vi "valve_VCH.vi"(4 "ZB01 (F)":bool, 6 "XB24 (F)":bool, 7 "Alarm":bool[](array[boolean])=[FALSE, FALSE], 10 "Z_control":T5={"Z_HSw"=1, "Z_HSetState"=enum."on (closed)", "Z_ASetState"=enum."on (closed)", "Z_DSetState"=enum."on (closed)"}, 11 "valve_VCH_in":refnum<class "valve_VCH.lvclass">) -> (1 "YB":bool[](array[boolean]), 2 "Z_out":T1={"Z_Source"=enum."local disabled", "Z_SetState"=enum."initialization", "Z_State"=enum."initialization", "Z_State_T"=0, "ZM_State"=enum."initialization", "ZM_State_T"=0, "ALR  L1"=FALSE, "ALR  L2"=FALSE, "HH_run"=0}, 3 "valve_VCH_in 2":refnum<class "valve_VCH.lvclass">)   [LabVIEW 2019, in "valve_VCH.lvclass"]
uses:
  valve_VCH.lvclass
  ctl/Z_control_VCH.ctl
  ctl/Z_State_VCH.ctl
  ctl/Z.ctl
  Heating/ctl/Z_source.ctl
  ctl/ZM_State_VCH.ctl
  valve_VCH.lvclass/valve_VCH.ctl
  ZM_state/valve_VCH_ZM_state.lvclass/valve_VCH_ZM_state.ctl
  Z_state/valve_VCH_Z_state.lvclass/valve_VCH_Z_state.ctl
  Sequence/State/State.lvclass/State.ctl
  Sequence/State/Read T (ms).vi
  Z_state/valve_VCH_Z_state.lvclass
  D:/my_projects/projects/Algorithms/Labview/19/Sequence/State/State.lvclass
  ZM_state/valve_VCH_ZM_state.lvclass
  Sequence/State/Step.vi
  Valves.lvlib
  Heating/Heating.lvlib
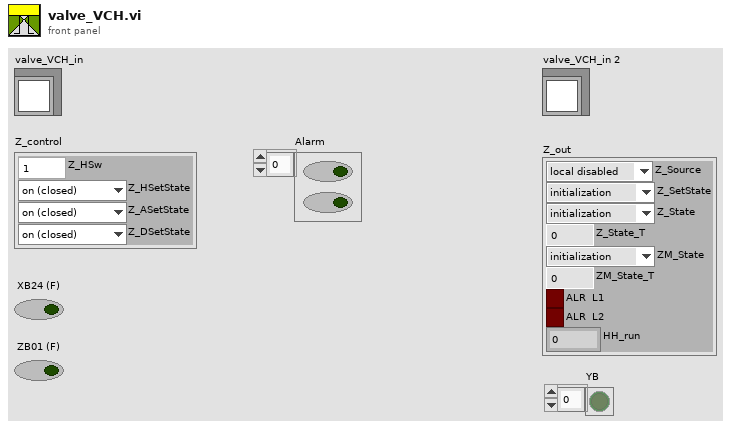
[diagram p1: front panel]
types:
  T1 = typedef "Valves.lvlib/Z.ctl" = cluster{"Z_Source":T2, "Z_SetState":T3, "Z_State":T3, "Z_State_T":u32, "ZM_State":T4, "ZM_State_T":u32, "ALR  L1":bool, "ALR  L2":bool, "HH_run":i32}
  T2 = typedef "Heating.lvlib/Z_source.ctl" = enum8{"initialize", "local disabled", "local hand", "hand", "auto", "dist"}
  T3 = typedef "Valves.lvlib/Z_State_VCH.ctl" = enum8{"initialization", "alarm", "disabled", "not ready", "closed ready", "reserv", "reserv1", "reserv2", "reserv3", "check", "on min", "open", "on (closed)"}
  T4 = typedef "Valves.lvlib/ZM_State_VCH.ctl" = enum8{"initialization", "closed", "big_pause", "little_pause", "open", "close_cmd"}
  T5 = typedef "Valves.lvlib/Z_control_VCH.ctl" = cluster{"Z_HSw":u8, "Z_HSetState":T3, "Z_ASetState":T3, "Z_DSetState":T3}
  T6 = cluster{"Z_Source":T2, "Z_Set_State":T3, "ZM_State":T4}
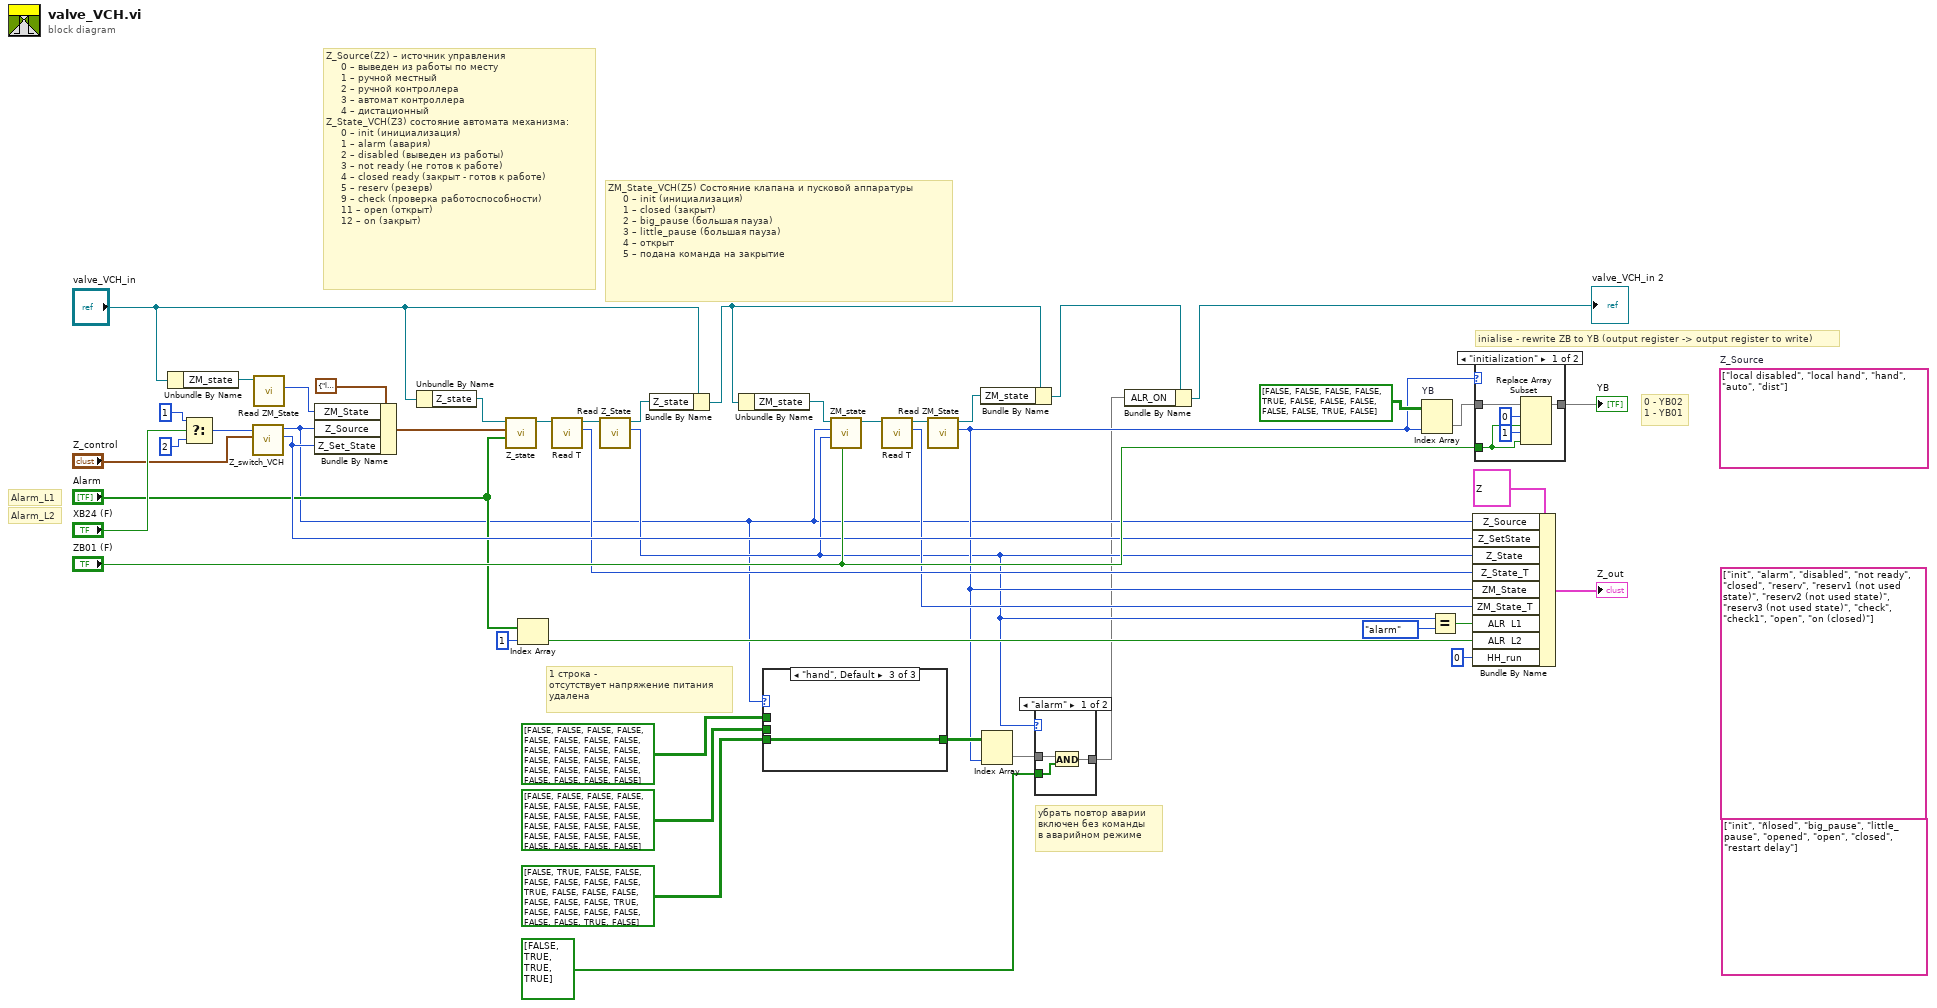
[diagram p0: block diagram]
diagram:
  (unwired) string[] ["init", "alarm", "disabled", "not ready", "closed", "reserv", "reserv1 (not used state)", "reserv2 (not used state)", "reserv3 (not used state)", "check", "check1", "open", "on (closed)"]
  (unwired) string[] ["local disabled", "local hand", "hand", "auto", "dist"]  # Z_Source
  (unwired) string[] ["init", "ñlosed", "big_pause", "little_pause", "opened", "open", "closed", "restart delay"]
  # "Alarm_L2"
  # "Alarm_L1"
  # "inialise - rewrite ZB to YB (output register -> output register to write)"
  # "0 - YB02\n1 - YB01"
  # "1 строка - \nотсутствует напряжение питания\nудалена"
  # "убрать повтор аварии\nвключен без команды\nв аварийном режиме"
  # "Z_Source(Z2) – источник управления\n     0 – выведен из работы по месту\n     1 – ручной местный\n     2 – ручной контроллера\n     3 – автомат контроллера\n     4 – дистационный\nZ_State_VCH(Z3) состояние автомата механизма:\n     0 – init (инициализация)\n     1 – alarm (авария)\n     2 – disabled (выведен из работы)\n     3 – not ready (не готов к работе)\n     4 – closed ready (закрыт - готов к работе)\n     5 – reserv (резерв)\n     9 – check (проверка работоспособности)\n     11 – open (открыт)\n     12 – on (закрыт)"
  # "ZM_State_VCH(Z5) Состояние клапана и пусковой аппаратуры\n     0 – init (инициализация)\n     1 – сlosed (закрыт)\n     2 – big_pause (большая пауза)\n     3 – little_pause (большая пауза)\n     4 – открыт\n     5 – подана команда на закрытие"
  n1 = Unbundle By Name("valve_VCH_in") -> ("ZM_state"=w11:refnum<class "valve_VCH_ZM_state.lvclass">)
  n2 = Select(t=u32 1, s="XB24 (F)", f=u32 2) -> (s? t:f=w43:u32)
  n3 = call "Z_switch_VCH.vi"("Z"="Z_control", "Z_LSw (2-auto)"=w43) -> ("Z_SetState"=w31:T3, "Z_Source"=w7:T2)  [unwired: 8 in]
  n4 = call "Read ZM_State.vi"("valve_VCH_ZM_state in"=w11) -> ("ZM_State_VCH"=w10:T4)  [unwired: 9 in, 1 out]
  n5 = Bundle By Name(cluster=T6 {"Z_Source"=enum."local disabled", "Z_Set_State"=enum."initialization", "ZM_State"=enum."initialization"} ("Z_In"), "ZM_State"=w10, "Z_Source"=w7, "Z_Set_State"=w31) -> (w23:T6)
  n6 = Unbundle By Name("valve_VCH_in") -> ("Z_state"=w3:refnum<class "valve_VCH_Z_state.lvclass">)
  n7 = call "Z_state.vi"("Alarm"="Alarm", "Z_In"=w23, "Z_state in"=w3) -> ("Z_state out"=w20:refnum<class "valve_VCH_Z_state.lvclass">)  [unwired: 8 in]
  n8 = Index Array(array="Alarm", index=1) -> (element=w26:bool)
  n9 = call "Read T.vi"("valve_VCH_Z_state in"=w20) -> ("T (ms)"=w21:u32, "valve_VCH_Z_state out"=w19:refnum<class "valve_VCH_Z_state.lvclass">)  [unwired: 9 in]
  n10 = call "Read Z_State.vi"("valve_VCH_Z_state in"=w19) -> ("Z_State_VCH"=w8:T3, "valve_VCH_Z_state out"=w18:refnum<class "valve_VCH_Z_state.lvclass">)  [unwired: 9 in]
  n11 = Bundle By Name(cluster="valve_VCH_in", "Z_state"=w18) -> (w13:refnum<class "valve_VCH.lvclass">)
  n12 = Unbundle By Name(w13) -> ("ZM_state"=w2:refnum<class "valve_VCH_ZM_state.lvclass">)
  n13 = case shown="\"hand\", Default" w7 {
    tunnel: bool[][] [[FALSE, FALSE, FALSE, FALSE, FALSE, FALSE], [FALSE, FALSE, FALSE, FALSE, FALSE, FALSE], [FALSE, FALSE, FALSE, FALSE, FALSE, FALSE], [FALSE, FALSE, FALSE, FALSE, FALSE, FALSE]] ("Array") -> [w47 _ _]
    tunnel: bool[][] [[FALSE, FALSE, FALSE, FALSE, FALSE, FALSE], [FALSE, FALSE, FALSE, FALSE, FALSE, FALSE], [FALSE, FALSE, FALSE, FALSE, FALSE, FALSE], [FALSE, FALSE, FALSE, FALSE, FALSE, FALSE]] ("Array") -> [_ w48 _]
    tunnel: bool[][] [[FALSE, TRUE, FALSE, FALSE, FALSE, FALSE], [FALSE, FALSE, TRUE, FALSE, FALSE, FALSE], [FALSE, FALSE, FALSE, TRUE, FALSE, FALSE], [FALSE, FALSE, FALSE, FALSE, TRUE, FALSE]] ("Array 3") -> [_ _ w49]
    tunnel: [w47 w48 w49] -> w40
    frame "initialize", "local disabled" {
    }
    frame "local hand" {
    }
    frame "hand", Default {
    }
  }
  n14 = call "ZM_state.vi"("ZB01"="ZB01 (F)", "Z_State"=w8, "Z_Source (hand)"=w7, "ZM_state in"=w2) -> ("ZM_state out"=w17:refnum<class "valve_VCH_ZM_state.lvclass">)  [unwired: 7 in]
  n15 = call "Read T.vi"("valve_VCH_ZM_state in"=w17) -> ("T (ms)"=w15:u32, "valve_VCH_ZM_state out"=w16:refnum<class "valve_VCH_ZM_state.lvclass">)  [unwired: 9 in]
  n16 = call "Read ZM_State.vi"("valve_VCH_ZM_state in"=w16) -> ("ZM_State_VCH"=w9:T4, "valve_VCH_ZM_state out"=w14:refnum<class "valve_VCH_ZM_state.lvclass">)  [unwired: 9 in]
  n17 = Bundle By Name(cluster=w13, "ZM_state"=w14) -> (w5:refnum<class "valve_VCH.lvclass">)
  n18 = Index Array(array=w40, index (col)=w9) -> (element=w38:bool[])  [unwired: 1 in]
  n19 = case shown="\"alarm\"" w8 {
    tunnel: bool[] [FALSE, TRUE, TRUE, TRUE] ("Array 4") -> [w51 _]
    tunnel: w38 -> [w52 w53]
    tunnel: [w50 w53] -> w6
    frame "alarm" {
      n20 = And(x=w52, y=w51) -> (x .and. y?=w50:bool[])
    }
    frame "disabled", Default {
    }
  }
  n21 = Bundle By Name(cluster=w5, "ALR_ON"=w6) -> (→"valve_VCH_in 2":refnum<class "valve_VCH.lvclass">)
  n22 = Index Array "YB"(array=bool[][] [[FALSE, FALSE, FALSE, FALSE, TRUE, FALSE], [FALSE, FALSE, FALSE, FALSE, TRUE, FALSE]] ("Array 5"), index (col)=w9) -> (element=w37:bool[])  [unwired: 1 in]
  n23 = Equal?(x=w8, y=Z_State_VCH."alarm") -> (x = y?=w28:bool)
  n24 = Bundle By Name(cluster=T1 {"Z_Source"=enum."local disabled", "Z_SetState"=enum."initialization", "Z_State"=enum."initialization", "Z_State_T"=0, "ZM_State"=enum."initialization", "ZM_State_T"=0, "ALR  L1"=FALSE, "ALR  L2"=FALSE, "HH_run"=0} ("Z"), "Z_Source"=w7, "Z_SetState"=w31, "Z_State"=w8, "Z_State_T"=w21, "ZM_State"=w9, "ZM_State_T"=w15, "ALR  L1"=w28, "ALR  L2"=w26, "HH_run"=0) -> (→"Z_out":T1)
  n25 = case shown="\"initialization\"" w9 {
    tunnel: w37 -> [w58 w59]
    tunnel: [w55 w59] -> w36
    tunnel: "ZB01 (F)" -> [w54 _]
    frame "initialization" {
      n26 = Replace Array Subset(array=w58, new element #1=w54, index #1=0 ("index"), new element #2=w54, index #2=1 ("index")) -> (w55:bool[])
    }
    frame "closed", Default {
    }
  }
  "YB" <- w36
